vi "_CSMOFGV Release.vi"(8 "Error in":errorcluster caption="Error in (no error)", 11 "CSMQ":T1={"Requested Name"="", "Module Name"="", "Mode"=enum."Stand Alone", "Queue"=refnum, "CSM-Data"=refnum, "User Event"=refnum, "Status Change Event"=refnum, "Allowed Messages"=[], "Mode-Data"=refnum, "Group Name"="", "Exit Event"=refnum}) -> (0 "Error out":errorcluster)   [LabVIEW 2020, in "Communicable State Machine.lvlib"]
uses:
  Communicable State Machine.lvlib
  _CSMObj.ctl
  Priority Queue.lvclass
  _CSM_MODE.ctl
  _CSMObj-Data.ctl
  _CSM Status Change Event Data.ctl
  _CSMObj-ModeData.ctl
  _CSMOFGVOPER.ctl
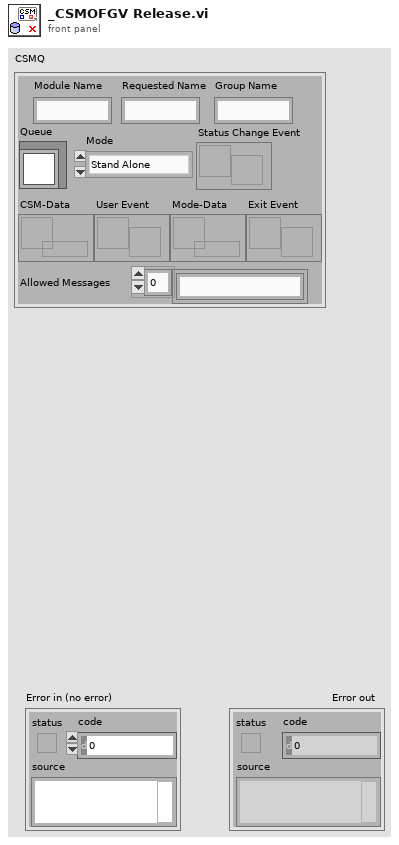
[diagram p1: front panel]
types:
  T1 = typedef "Communicable State Machine.lvlib/_CSMObj.ctl" = cluster{"Requested Name":string, "Module Name":string, "Mode":T2, "Queue":refnum<class "Priority Queue.lvclass">, "CSM-Data":refnum<data-value>, "User Event":refnum<user-event>, "Status Change Event":refnum<user-event>, "Allowed Messages":string[], "Mode-Data":refnum<data-value>, "Group Name":string, "Exit Event":refnum<user-event>}
  T2 = typedef "Communicable State Machine.lvlib/_CSM_MODE.ctl" = enum16{"Not Exist", "Stand Alone", "CSM", "Worker Agent", "Worker", "Chain", "Chain Node"}
  T3 = typedef "Communicable State Machine.lvlib/_CSMOFGVOPER.ctl" = enum16{"Create If not Exist", "Get By Name", "List", "Check If Name Exists", "Release", "Module Status", "Create Status Event Handler", "Destroy Status Event Handler"}
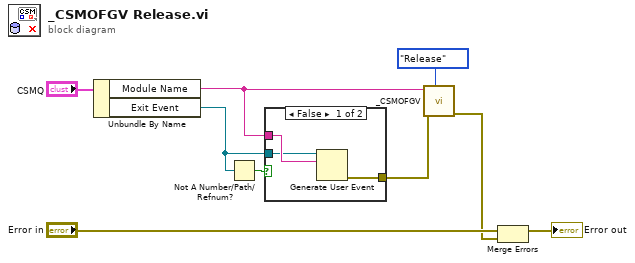
[diagram p0: block diagram]
diagram:
  n1 = Unbundle By Name("CSMQ") -> ("Module Name"=w4:string, "Exit Event"=w2:refnum<user-event>)
  n2 = Not A Number/Path/Refnum?(number/path/refnum=w2) -> (NaN/Path/Refnum?=w1:bool)
  n3 = case shown="False" w1 {
    tunnel: w4 -> [w12 _]
    tunnel: [w11 _] -> w3
    tunnel: w2 -> [w10 _]
    frame False {
      n4 = Generate User Event(user event=w10, event data cluster=w12) -> (error out=w11:errorcluster)  [unwired: 2 in, 1 out]
    }
    frame True {
    }
  }
  n5 = call "_CSMOFGV.vi"("Operation"=_CSMOFGVOPER."Release", "Error in"=w3, "Name(\"\" to use uuid) in"=w4) -> ("Error out"=w5:errorcluster)  [unwired: 6 in, 2 out]
  n6 = Merge Errors("Error in", w5) -> (→"Error out":errorcluster)
